vi "User Interface.vi"(8 "error in (no error)":errorcluster, 11 "User Interface in":refnum<class "User Interface.lvclass">) -> (0 "error out":errorcluster, 3 "User Interface out":refnum<class "User Interface.lvclass">)   [LabVIEW 2017, in "PXImc.lvlib" / "Thread User Interface.lvclass"]
uses:
  Thread User Interface.lvclass
  DSF Core.lvlibp/Classes/User Interface/User Interface.lvclass
  Configurations/Thread/Thread Configuration.lvclass
  Configurations/Thread/Thread Configuration.lvclass/Thread Configuration.ctl
  C:/Git/DSF/Components/DSF Core.lvlibp/Classes/Configuration/Configuration.lvclass
panel:
  in  "Interface":string
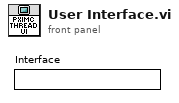
[diagram p1: front panel]
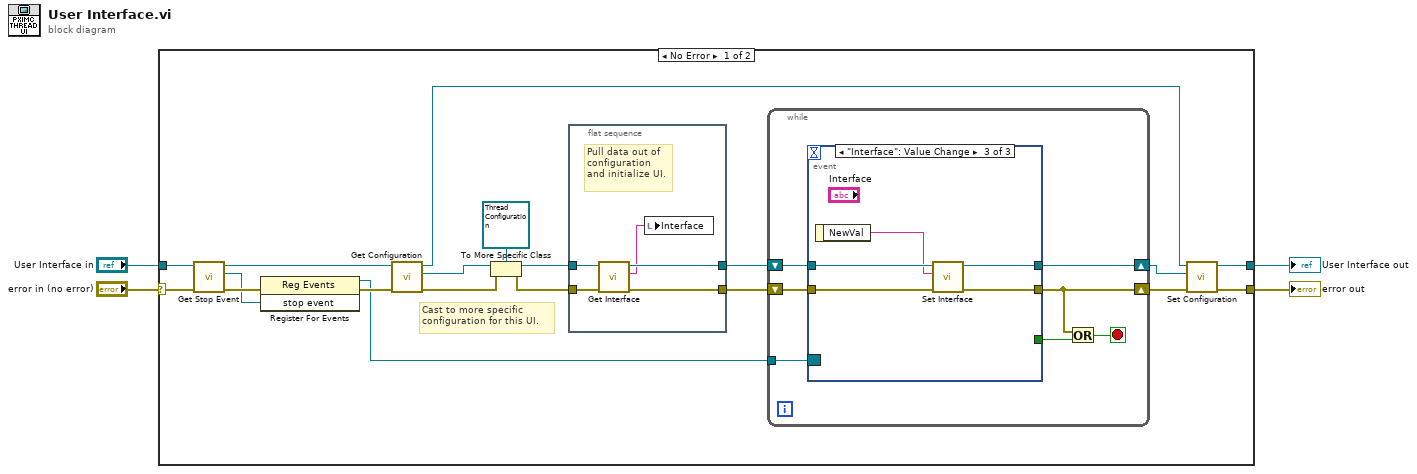
[diagram p0: block diagram]
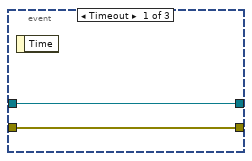
[diagram p2: hidden frame]
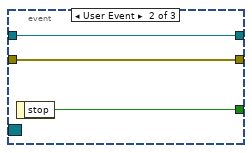
[diagram p3: hidden frame]
diagram:
  n1 = case shown="No Error" "error in (no error)" {
    selector: "error in (no error)" -> [w19 w47]
    tunnel: [w7 w47] -> w4
    tunnel: "User Interface in" -> [w18 w46]
    tunnel: [w6 w46] -> w1
    frame No Error {
      # "Cast to more specific configuration for this UI."
      n2 = call "Get Stop Event.vi"("error in (no error)"=w19, "User Interface in"=w18) -> ("error out"=w17:errorcluster, "stop event"=w16:refnum<user-event>, "User Interface out"=w15:refnum<class "User Interface.lvclass">)  [unwired: 7 in]
      n3 = register-events(error in=w17, w16) -> (reference out=w13:refnum<event-registration>, error out=w14:errorcluster)  [unwired: 1 in]
      n4 = call "Get Configuration.vi"("error in (no error)"=w14, "User Interface in"=w15) -> ("error out"=w12:errorcluster, "configuration"=w10:refnum<class "Configuration.lvclass">, "User Interface out"=w5:refnum<class "User Interface.lvclass">)  [unwired: 7 in]
      n5 = To More Specific Class(target class=refnum<class "Thread Configuration.lvclass"> refnum ("Configuration out"), reference=w10, error in=w12) -> (specific class reference=w23:refnum<class "Thread Configuration.lvclass">, error out=w20:errorcluster)
      n6 = flat-sequence {
        tunnel: [w25] -> w21
        tunnel: w20 -> [w28]
        tunnel: w23 -> [w27]
        tunnel: [w26] -> w22
        frame #0 {
          # "Pull data out of configuration and initialize UI."
          n7 = call "Get Interface.vi"("error in (no error)"=w28, "Thread Configuration in"=w27) -> ("error out"=w25:errorcluster, "interface"=w24:tag, "Thread Configuration out"=w26:refnum<class "Thread Configuration.lvclass">)  [unwired: 7 in]
          n8 = local write "Interface"(w24) -> ()
        }
      }
      n9 = while {
        tunnel: w13 -> [w35]
        shift-right: [w33] -> w8
        shift-left: w21 -> [w34]
        shift-right: [w29] -> w9
        shift-left: w22 -> [w30]
        stop <- w32 stop-if-true
        n10 = event shown="[2] \"Interface\": Value Change" {
          selector: w35 -> [_ _ _]
          dyn-events: _ -> [_ _ _]
          timeout: _ -> [_ _ _]
          tunnel: [_ w38 _] -> w31
          tunnel: w34 -> [w37 w40 w45]
          tunnel: [w37 w40 w41] -> w33
          tunnel: w30 -> [w36 w39 w44]
          tunnel: [w36 w39 w42] -> w29
          event Timeout {
            n11 = event-data() -> ()  [unwired: 1 in, 1 out]
          }
          event User Event {
            n12 = event-data() -> ("stop"=w38:bool)  [unwired: 1 in]
          }
          event "Interface": Value Change {
            n13 = event-data() -> ("NewVal"=w43:string)  [unwired: 1 in]
            n14 = call "Set Interface.vi"("error in (no error)"=w45, "interface"=w43, "Thread Configuration in"=w44) -> ("error out"=w41:errorcluster, "Thread Configuration out"=w42:refnum<class "Thread Configuration.lvclass">)  [unwired: 7 in]
          }
        }
        n15 = Or(x=w33, y=w31) -> (x .or. y?=w32:bool)
      }
      n16 = call "Set Configuration.vi"("error in (no error)"=w8, "configuration"=w9, "User Interface in"=w5) -> ("error out"=w7:errorcluster, "User Interface out"=w6:refnum<class "User Interface.lvclass">)  [unwired: 7 in]
    }
    frame Error {
    }
  }
  "error out" <- w4
  "User Interface out" <- w1
